vi "SetTraverse.vi"(8 "error in (no error)":errorcluster, 10 "Traverse":bool, 11 "VariantTree in":refnum<class "Failures_VariantTree__VP.lvclass">) -> (0 "error out":errorcluster, 3 "VariantTree out":refnum<class "Failures_VariantTree__VP.lvclass">)   [LabVIEW 2013, in "Failures_VariantTree__VP.lvclass"]
uses:
  Failures_VariantTree__VP.lvclass
  Failures_VariantTree__VP.lvclass/Failures_VariantTree__VP.ctl
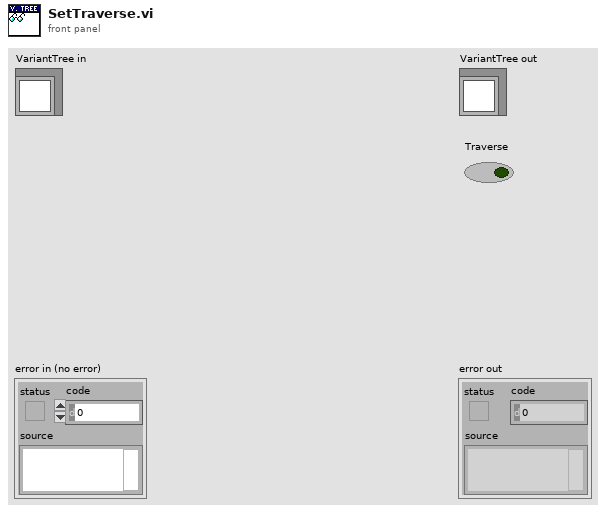
[diagram p1: front panel]
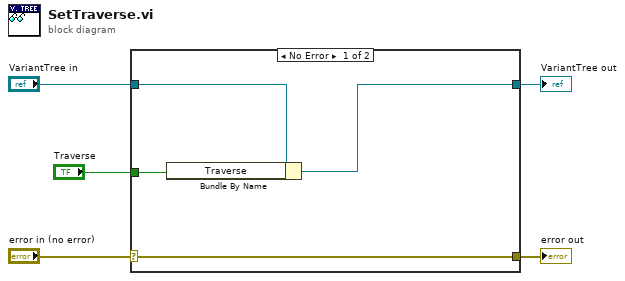
[diagram p0: block diagram]
diagram:
  n1 = case shown="No Error" "error in (no error)" {
    selector: "error in (no error)" -> [w9 w10]
    tunnel: [w9 w10] -> w4
    tunnel: [w6 w11] -> w2
    tunnel: "VariantTree in" -> [w7 w11]
    tunnel: "Traverse" -> [w8 _]
    frame No Error {
      n2 = Bundle By Name(cluster=w7, "Traverse"=w8) -> (w6:refnum<class "Failures_VariantTree__VP.lvclass">)
    }
    frame Error {
    }
  }
  "error out" <- w4
  "VariantTree out" <- w2
